vi "tool.vi"() -> ()   [LabVIEW 2015]
panel:
  in  "String":string
  out "x > y?":bool
  in  "OK Button":bool
  in  "stop":bool
  out "Numeric":i32
  out "number (0 to 1)":dbl
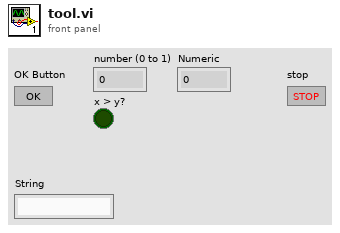
[diagram p1: front panel]
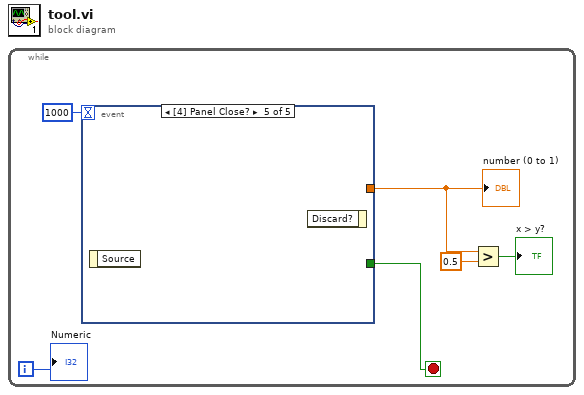
[diagram p0: block diagram]
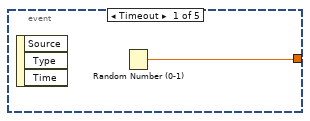
[diagram p2: hidden frame]
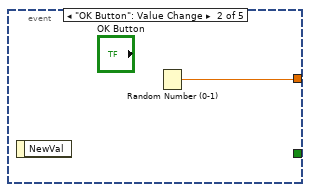
[diagram p3: hidden frame]
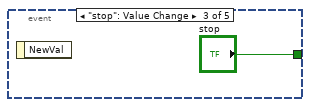
[diagram p4: hidden frame]
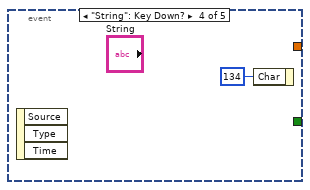
[diagram p5: hidden frame]
diagram:
  n1 = while {
    i -> [w5]
    stop <- w4 stop-if-true
    n2 = event shown="[4] Panel Close?" {
      selector: _ -> [_ _ _ _ _]
      dyn-events: _ -> [_ _ _ _ _]
      timeout: 1000 -> [_ _ _ _ _]
      tunnel: [_ _ "stop" _ _] -> w4
      tunnel: [w7 w8 _ _ _] -> w3
      event Timeout {
        n3 = event-data() -> ()  [unwired: 1 in, 3 out]
        n4 = Random Number (0-1)() -> (number: 0 to 1=w7:dbl)
      }
      event "OK Button": Value Change {
        n5 = event-data() -> ()  [unwired: 1 in, 1 out]
        n6 = Random Number (0-1)() -> (number: 0 to 1=w8:dbl)
      }
      event "stop": Value Change {
        n7 = event-data() -> ()  [unwired: 1 in, 1 out]
      }
      event "String": Key Down? {
        n8 = event-data() -> ()  [unwired: 1 in, 3 out]
        n9 = event-data("Char"=i16 134) -> ()  [unwired: 1 in, 1 out]
      }
      event Panel Close? {
        n10 = event-data() -> ()  [unwired: 1 in, 1 out]
        n11 = event-data() -> ()  [unwired: 2 in, 1 out]
      }
    }
    "number (0 to 1)" <- w3
    n12 = Greater?(x=w3, y=0.5) -> (0:→"x > y?":bool)
    "Numeric" <- w5
  }
